vi "CAN Read.vi"(4 "interface":refnum<k21>) -> (2 "data 2":T1[](array[typedef]) {"payload" format="%x"; "timestamp" format="%<%.7X\n%x>T"; "type" items=["CAN Data"=0, "CAN Remote"=1, "CAN Bus Error"=2, "CAN 2.0 Data"=8, "CAN FD Data"=16, "CAN FD+BRS Data"=24, "J1939 Data"=192, "Delay"=224, "Log Trigger"=225, "Start Trigger"=226]; "identifier" format="%x"})   [LabVIEW 2022 SP3]
uses:
  <vilib>/xnet/xnet.llb/XNET Frame CAN.ctl
  <vilib>/xnet/xnet.llb/XNET Frame Type CAN.ctl
  <vilib>/xnet/xnet.llb/XNET Control Scope.ctl
  <vilib>/xnet/xnet.llb/XNET Create Session (Frame Input Stream).vi
  <vilib>/xnet/xnet.llb/XNET Read (Frame CAN).vi
  <resource>/objmgr/xnet.rc
panel:
  in  "stop":bool
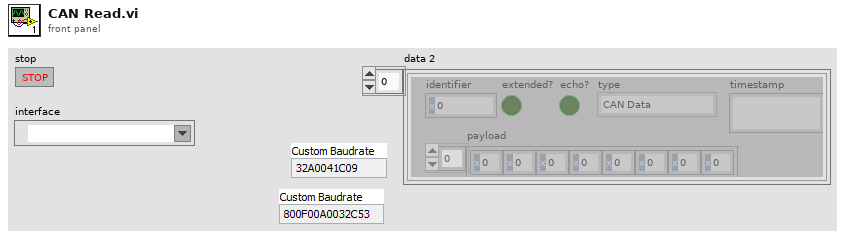
[diagram p1: front panel]
types:
  T1 = typedef "XNET Frame CAN.ctl" = cluster{"timestamp":timestamp, "payload":u8[], "identifier":u32, "type":T2, "extended?":bool, "echo?":bool}
  T2 = typedef "XNET Frame Type CAN.ctl" = u8
  T3 = typedef "XNET Control Scope.ctl" = u32
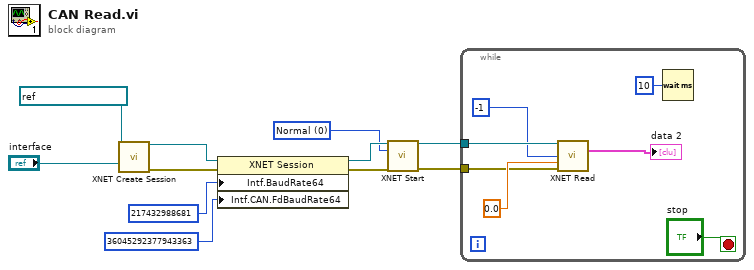
[diagram p0: block diagram]
diagram:
  w4 = T3 0 items=["Normal", "Session Only", "Interface Only", "Session Only Blocking"] ("scope (normal)")
  n1 = call-poly <vilib>:"XNET Create Session.vi"("cluster (:memory:)"=refnum<k21> "Elatch_Labview", "interface"="interface") -> ("session out"=w8:refnum<k21>, "error out"=w9:errorcluster)  [unwired: 12 in]
  n2 = property class="XNET Session"(reference=w8, error in=w9, "Intf.BaudRate64"=u64 217432988681 ("Interface:64bit Baud Rate"), "Intf.CAN.FdBaudRate64"=u64 36045292377943363 ("Interface:CAN:64bit FD Baud Rate")) -> (reference out=w6:refnum<k21>, error out=w5:errorcluster)
  n3 = call <vilib>:"XNET Start.vi"("session in"=w6, "scope (normal)"=w4, "error in (no error)"=w5) -> ("session out"=w2:refnum<k21>, "error out"=w1:errorcluster)  [unwired: 11 in]
  n4 = while {
    tunnel: w2 -> [w17]
    tunnel: w1 -> [w14]
    stop <- "stop" stop-if-true
    n5 = call-poly <vilib>:"XNET Read.vi"("session in"=w17, "number to read (-1)"=-1, "timeout (0)"=0.0, "error in (no error)"=w14) -> ("data"=→"data 2":T1[])  [unwired: 8 in, 3 out]
    n6 = Wait (ms)(milliseconds to wait=u32 10) -> ()  [unwired: 1 out]
  }
